vi "Write Settings to file.vi"(8 "error in (no error)":errorcluster, 10 "settings":T1, 11 "Refnum in":T2) -> (0 "error out":errorcluster, 2 "settings id":string, 3 "Refnum out":T2)   [LabVIEW 2017, in "Data Sharing Framework Engine.lvlib"]
uses:
  Data Sharing Framework Engine.lvlib
  Configuration/1.0.0/Public/Controls/DSF Config Data RefNum.ctl
  Configuration/1.0.0/Public/Controls/DSF Settings Info.ctl
  Configuration/1.0.0/Public/Write Item/Write Settings.vi
  Configuration/1.0.0/Data Sharing Framework Configuration.lvlib
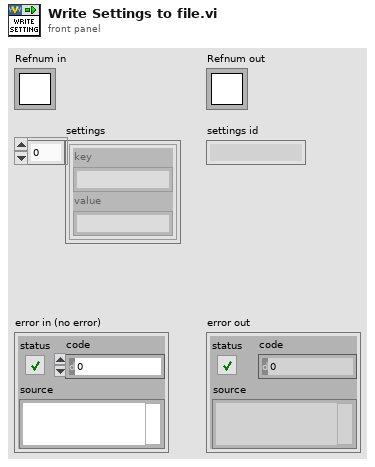
[diagram p1: front panel]
types:
  T1 = typedef "Data Sharing Framework Configuration.lvlib/DSF Settings Info.ctl" = cluster{"key":string, "value":string}[]
  T2 = typedef "Data Sharing Framework Configuration.lvlib/DSF Config Data RefNum.ctl" = refnum<k1>
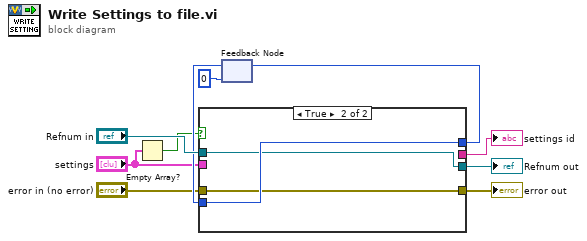
[diagram p0: block diagram]
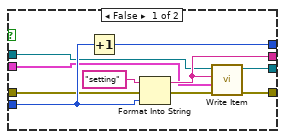
[diagram p2: hidden frame]
diagram:
  n1 = Empty Array?(array="settings") -> (empty?=w3:bool)
  n2 = feedback #1(0) -> (w6:i32)
  n3 = case shown="True" w3 {
    tunnel: [w19 w23] -> w7
    tunnel: w6 -> [w18 w23]
    tunnel: [w17 _] -> w8
    tunnel: "settings" -> [w16 _]
    tunnel: "Refnum in" -> [w15 w22]
    tunnel: [w14 w22] -> w10
    tunnel: "error in (no error)" -> [w13 w21]
    tunnel: [w11 w21] -> w1
    frame False {
      n4 = Increment(x=w18) -> (x+1=w19:i32)
      n5 = Format Into String(initial string="setting", error in=w13, w18) -> (resulting string=w17:string, error out=w12:errorcluster)  [unwired: 1 in]
      n6 = call-poly "Write Item.vi"("error in (no error)"=w12, "settings values"=w16, "id"=w17, "dsf refnum"=w15) -> ("error out"=w11:errorcluster, "dsf refnum out"=w14:T2)  [unwired: 5 in, 1 out]
    }
    frame True {
    }
  }
  "Refnum out" <- w10
  "settings id" <- w8
  "error out" <- w1
  n7 = feedback-in #1(w7) -> ()
